vi "arangeIdx.vi"(9 "Offset":i32, 11 "Number":i32) -> (3 "Idx Array":i32[](array[numeric]))   [LabVIEW 2016]
doc: "Get the index array from offset value to specified integer. The default value of offset is 0."
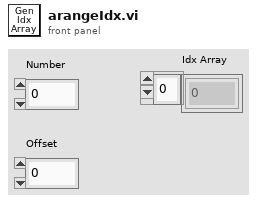
[diagram p1: front panel]
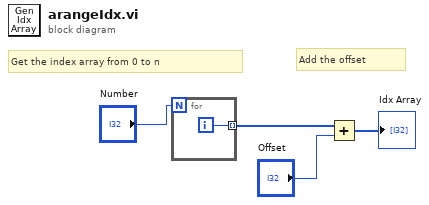
[diagram p0: block diagram]
diagram:
  # "Add the offset"
  # "Get the index array from 0 to n"
  n1 = for {
    N: "Number" -> [_]
    tunnel: [w5] -> w3 mode=indexing
    i -> [w5]
  }
  n2 = Add(x=w3, y="Offset") -> (x+y=→"Idx Array":i32[])
